vi "Obtain Header.vi"(8 "error in (no error)":errorcluster, 11 "GUID":string) -> (0 "error out":errorcluster, 3 "Linked List Header out":refnum<class "Linked List Header.lvclass">)   [LabVIEW 2019, in "Linked Lists.lvlib" / "Linked List Header.lvclass"]
uses:
  <vilib>/gpm_packages/@cs/linked-list/Source/Linked List/Linked List Header/Linked List Header.lvclass
  <vilib>/gpm_packages/@cs/lookup-table/Source/LookupTable/LookupTable.lvclass/LookupTable.ctl
  <vilib>/gpm_packages/@cs/linked-list/Source/Linked List/Linked List Header/Linked List Header.lvclass/Linked List Header.ctl
  bae55848-a840-4482-a4df-932c9ed6f776.vi
  <vilib>/gpm_packages/@cs/lookup-table/Source/LookupTable/Read Table Reference.vi
  bae55848-a840-4482-a4df-932c9ed6f776.vi/72e8528f-f6a8-432b-9e6f-bbd7709f9a19.vi
  <vilib>/gpm_packages/@cs/lookup-table/Source/LookupTable/LookupTable.lvclass
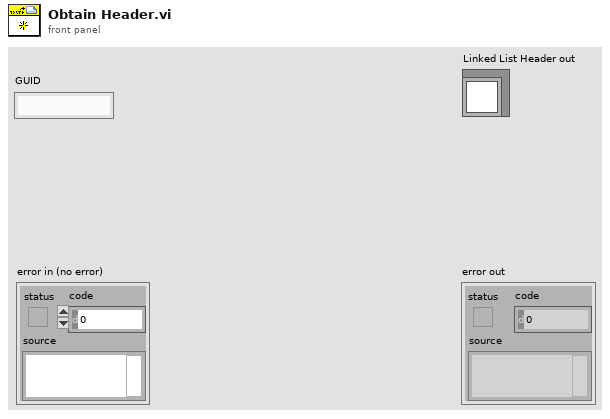
[diagram p1: front panel]
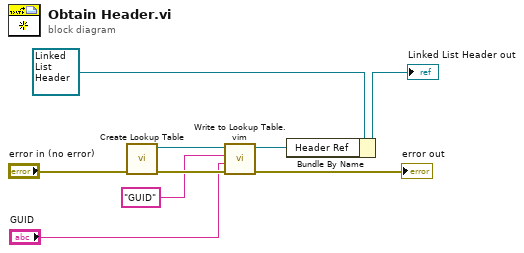
[diagram p0: block diagram]
diagram:
  n1 = call <vilib>:"Create Lookup Table.vi"("error in (no error)"="error in (no error)") -> ("error out"=w4:errorcluster, "LookupTable Reference"=w7:refnum<data-value>)  [unwired: 9 in]
  n2 = call "Write to Lookup Table.vim"("error in (no error)"=w4, "Item"="GUID", "Item Name"="GUID", "LookupTable Reference"=w7) -> ("error out"=→"error out":errorcluster, "LookupTable Reference Out"=w6:refnum<data-value>)  [unwired: 5 in, 1 out]
  n3 = Bundle By Name(cluster=refnum<class "Linked List Header.lvclass"> refnum ("Linked List Header in"), "Header Ref"=w6) -> (→"Linked List Header out":refnum<class "Linked List Header.lvclass">)
